vi "brc_daq_get_version.vi"() -> (3 "dll path":path)   [LabVIEW 2019, in "BRC-DAQ.lvlib"]
uses:
  BRC-DAQ.lvlib
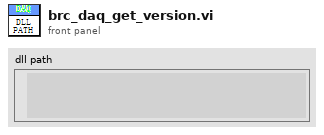
[diagram p1: front panel]
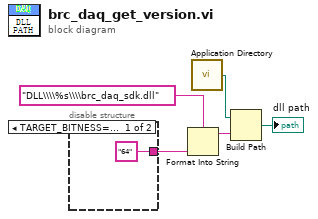
[diagram p0: block diagram]
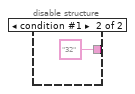
[diagram p2: hidden frame]
diagram:
  n1 = disable-structure shown="TARGET_BITNESS==64" {
    disable-tunnel: ["64" "32"] -> w2
    frame condition #0 (active) {
    }
    frame condition #1 {
    }
  }
  n2 = Format Into String(format string="DLL\\\\%s\\\\brc_daq_sdk.dll" ("名称或相对路径"), w2) -> (resulting string=w1:string)  [unwired: 2 in, 1 out]
  n3 = call <vilib>:"Application Directory.vi"() -> ("Application Directory"=w5:path)
  n4 = Build Path(base path=w5, name or relative path=w1) -> (appended path=→"dll path":path)
